vi "SwerveCalc.vi"(0 "Jx":dbl, 1 "Jy":dbl, 2 "Jr":dbl, 6 "Length":dbl=24.5, 7 "Width":dbl=24.5, 10 "MaxV":dbl) -> (20 "V0":dbl, 21 "V1":dbl, 22 "V2":dbl, 23 "V3":dbl, 24 "A0":dbl, 25 "A1":dbl, 26 "A2":dbl, 27 "A3":dbl)   [LabVIEW 2020]
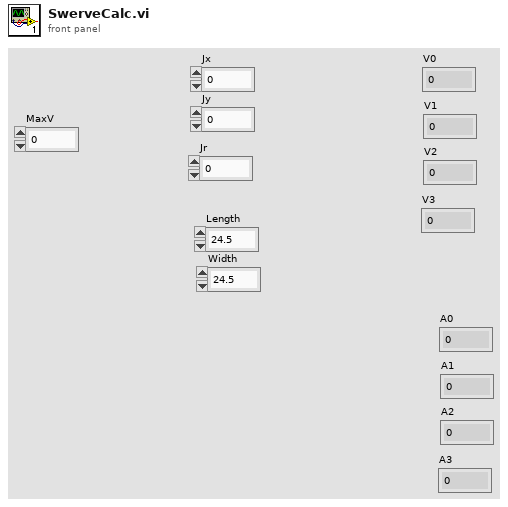
[diagram p1: front panel]
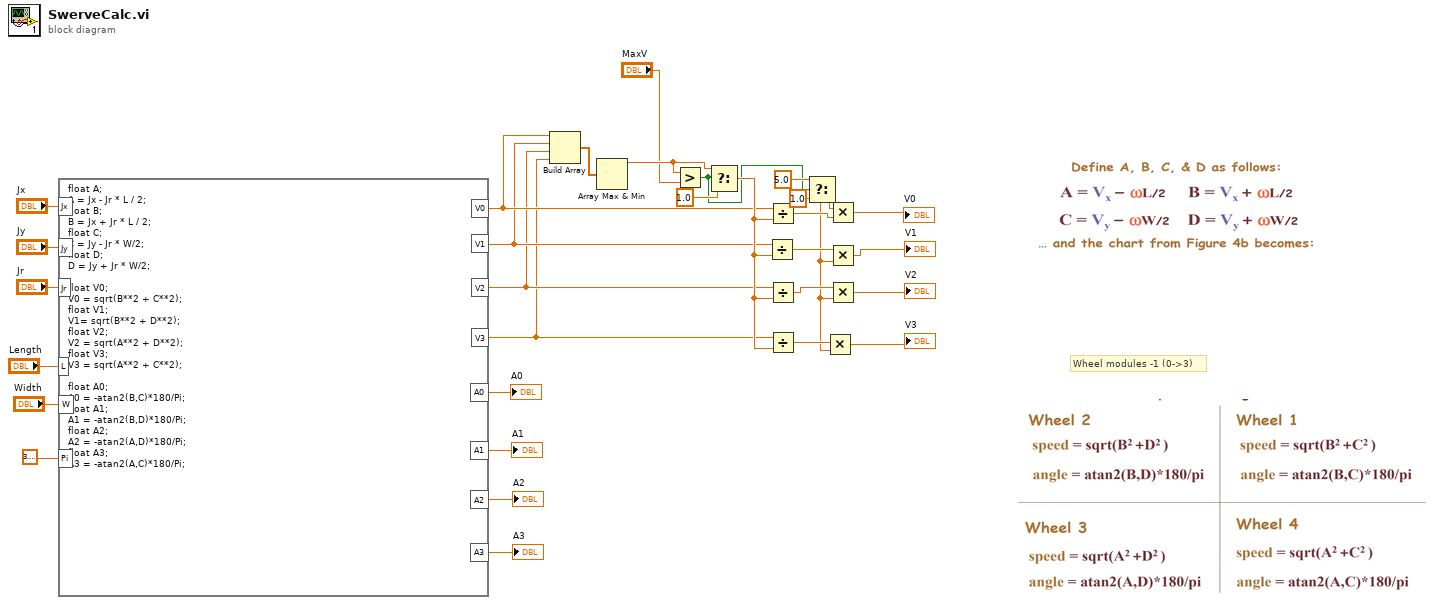
[diagram p0: block diagram]
diagram:
  # "Wheel modules -1 (0->3)"
  n1 = formula code="float A;\nA = Jx - Jr * L / 2;\nfloat B;\nB = Jx + Jr * L / 2;\nfloat C;\nC = Jy - Jr * W/2;\nfloat D;\nD = Jy + Jr * W/2;\n\nfloat V0;\nV0 = sqrt(B**2 + C**2);\nfloat V1;\nV1= sqrt(B**2 + D**2);\nfloat V2;\nV2 = sqrt(A**2 + D**2);\nfloat V3;\nV3 = sqrt(A**2 + C**2);\n\nfloat A0;\nA0 = -atan2(B,C)*180/Pi;\nfloat A1;\nA1 = -atan2(B,D)*180/Pi;\nfloat A2;\nA2 = -atan2(A,D)*180/Pi;\nfloat A3;\nA3 = -atan2(A,C)*180/Pi;"("Jx"="Jx", "Jy"="Jy", "Jr"="Jr", "L"="Length", "W"="Width", "Pi"=3.141592653589793) -> ("V0"=w18:dbl, "V1"=w17:dbl, "V2"=w16:dbl, "V3"=w15:dbl, "A0"=→"A0":dbl, "A1"=→"A1":dbl, "A2"=→"A2":dbl, "A3"=→"A3":dbl)
  n2 = Build Array(w18, w17, w16, w15) -> (w20:dbl[])
  n3 = Array Max & Min(array=w20) -> (max value=w21:dbl)  [unwired: 3 out]
  n4 = Greater?(x=w21, y="MaxV") -> (0:w1:bool)
  n5 = Select(t=w21, s=w1, f=1.0) -> (s? t:f=w19:dbl)
  n6 = Divide(x=w17, y=w19) -> (x/y=w9:dbl)
  n7 = Divide(x=w18, y=w19) -> (x/y=w10:dbl)
  n8 = Divide(x=w16, y=w19) -> (x/y=w8:dbl)
  n9 = Divide(x=w15, y=w19) -> (x/y=w7:dbl)
  n10 = Select(t=5.0, s=w1, f=1.0) -> (s? t:f=w6:dbl)
  n11 = Multiply(x=w7, y=w6) -> (x*y=→"V3":dbl)
  n12 = Multiply(x=w6, y=w10) -> (x*y=→"V0":dbl)
  n13 = Multiply(x=w9, y=w6) -> (x*y=→"V1":dbl)
  n14 = Multiply(x=w8, y=w6) -> (x*y=→"V2":dbl)
